vi "Matrix Multiply.vi"(9 "Vector":sgl[](array[numeric]), 11 "Matrix":sgl[][](array[numeric])) -> (3 "Product":sgl[](array[numeric]))   [LabVIEW 2020, in "3D Plot.lvclass"]
uses:
  3D Plot.lvclass
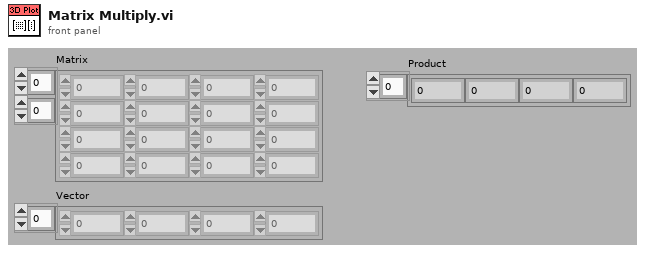
[diagram p1: front panel]
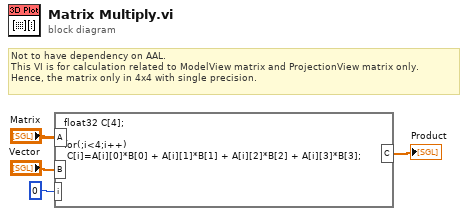
[diagram p0: block diagram]
diagram:
  # "Not to have dependency on AAL.\nThis VI is for calculation related to ModelView matrix and ProjectionView matrix only.\nHence, the matrix only in 4x4 with single precision."
  n1 = formula code="float32 C[4];\n\nfor(;i<4;i++)\n C[i]=A[i][0]*B[0] + A[i][1]*B[1] + A[i][2]*B[2] + A[i][3]*B[3];"("A"="Matrix", "B"="Vector", "i"=0 ("input variable")) -> ("C"=→"Product":sgl[])
